vi "Read BBM Slot.vi"(8 "error in (no error)":errorcluster, 9 "Slot Number":u32, 10 "Chuck Number":u32, 11 "WorkTable Class in":refnum<class "WorkTable Class.lvclass">) -> (0 "error out":errorcluster, 2 "BBM Slot":T1, 3 "WorkTable Class out":refnum<class "WorkTable Class.lvclass">)   [LabVIEW 2011, in "WorkTable Class.lvclass"]
uses:
  WorkTable Class.lvclass
  Type Definitions/Worktable_BBM Slot.ctl
  Vec3d Class/Vec3d Class.lvclass
  Orient3d Class/Orient3d Class.lvclass
  Utils/Type Definitions/Position_Orientation.ctl
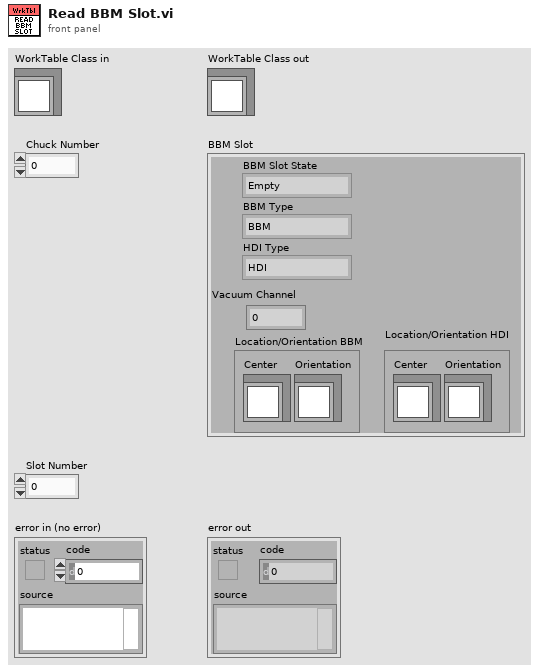
[diagram p1: front panel]
types:
  T1 = typedef "Worktable_BBM Slot.ctl" = cluster{"BBM Slot State":enum16{"Empty", "Unglued", "Stamped", "PartOnTop", "Weighted", "Unpotted", "Potted"}, "BBM Type":enum16{"BBM", "GlassSlide"}, "HDI Type":enum16{"HDI", "Polyimide"}, "Vacuum Channel":u8, "Location/Orientation BBM":T2, "Location/Orientation HDI":T2}
  T2 = typedef "Position_Orientation.ctl" = cluster{"Center":refnum<class "Vec3d Class.lvclass">, "Orientation":refnum<class "Orient3d Class.lvclass">}
  T3 = cluster{"BBM Chucks":cluster{"BBM Slots":T1[]}[]}
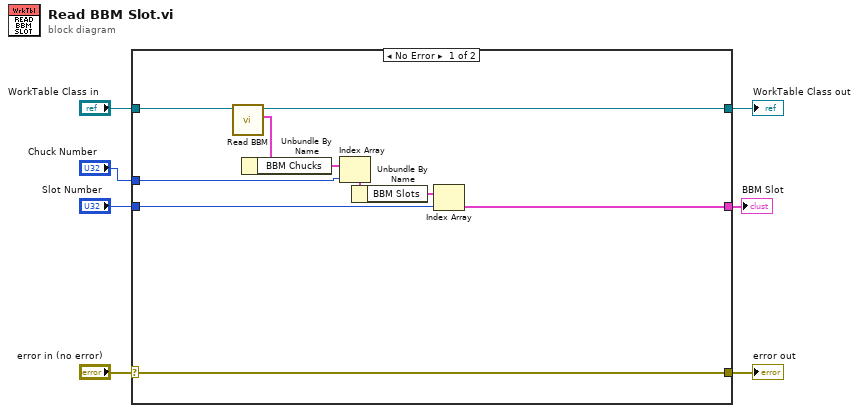
[diagram p0: block diagram]
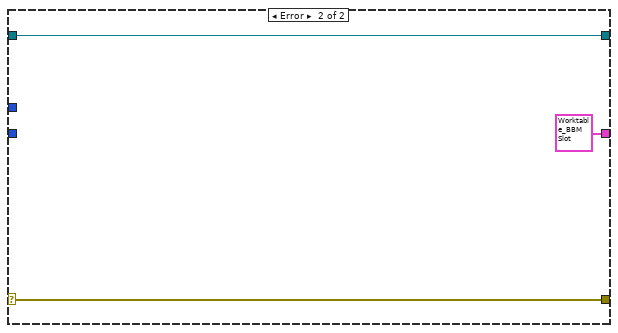
[diagram p2: hidden frame]
diagram:
  n1 = case shown="No Error" "error in (no error)" {
    selector: "error in (no error)" -> [w17 w20]
    tunnel: [w17 w20] -> w6
    tunnel: [w8 w19] -> w4
    tunnel: "WorkTable Class in" -> [w12 w19]
    tunnel: "Chuck Number" -> [w11 _]
    tunnel: "Slot Number" -> [w10 _]
    tunnel: [w9 T1 {"BBM Slot State"=enum."Empty", "BBM Type"=enum."BBM", "HDI Type"=enum."HDI", "Vacuum Channel"=0, "Location/Orientation BBM"={"Center"=refnum, "Orientation"=refnum}, "Location/Orientation HDI"={"Center"=refnum, "Orientation"=refnum}} ("BBM Slot")] -> w1
    frame No Error {
      n2 = call-dynamic "Read BBM.vi"("WorkTable in"=w12) -> ("BBM"=w13:T3, "WorkTable out"=w8:refnum<class "WorkTable Class.lvclass">)  [unwired: 8 in, 1 out]
      n3 = Unbundle By Name(w13) -> ("BBM Chucks"=w14:cluster{"BBM Slots":T1[]}[])
      n4 = Index Array(array=w14, index=w11) -> (element=w15:cluster{"BBM Slots":T1[]})
      n5 = Unbundle By Name(w15) -> ("BBM Slots"=w16:T1[])
      n6 = Index Array(array=w16, index=w10) -> (element=w9:T1)
    }
    frame Error {
    }
  }
  "error out" <- w6
  "WorkTable Class out" <- w4
  "BBM Slot" <- w1
